vi "_check_error.vi"(8 "error in (no error)":errorcluster, 11 "VISA resource name":refnum<visa-resource-name>) -> (0 "error out":errorcluster, 3 "VISA resource name out":refnum<visa-resource-name>)   [LabVIEW 2015, in "Rohde&Schwarz CMXP Base.lvlib"]
doc: "This VI checks for an error by sending *STB? query to the instrument. If the bit 2 (0x04) is set, it sends multiple SYST:ERR? queries to the instrument until the error query is empty."
uses:
  <instrlib>/Rohde&Schwarz CMXP Base/Rohde&Schwarz CMXP Base.lvlib
  <instrlib>/Rohde&Schwarz CMXP Base/Private/rsidr_core.llb/type_Attribute.ctl
  <instrlib>/Rohde&Schwarz CMXP Base/Private/rsidr_core.llb/type_Attribute_Data_Type.ctl
  <instrlib>/Rohde&Schwarz CMXP Base/Private/rsidr_core.llb/type_ReadWriteAccess.ctl
  <instrlib>/Rohde&Schwarz CMXP Base/Private/rsidr_core.llb/rsidr_core.lvlib
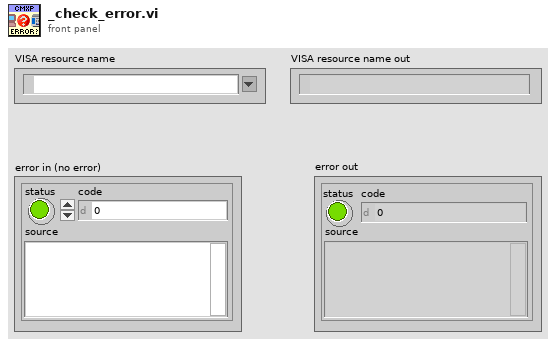
[diagram p1: front panel]
types:
  T1 = typedef "Rohde&Schwarz CMXP Base.lvlib/rsidr_core.lvlib/type_Attribute.ctl" = cluster{"Identifier":string, "Descriptive Name":string, "Data Type":T2, "Command":string, "Access":T3, "Range Table":string, "Read Callback":string, "Write Callback":string, "Supported Models":string, "Instrument Options":string, "Index":i32, "OPC Wait":bool, "No Status Check":bool, "Cache Only":bool}
  T2 = typedef "Rohde&Schwarz CMXP Base.lvlib/rsidr_core.lvlib/type_Attribute_Data_Type.ctl" = enum16{"Integer 32", "Double", "String", "Boolean", "None", "Integer 64", "RawString"}
  T3 = typedef "Rohde&Schwarz CMXP Base.lvlib/rsidr_core.lvlib/type_ReadWriteAccess.ctl" = enum16{"Read Only", "Write Only", "Read/Write"}
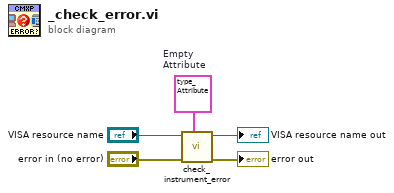
[diagram p0: block diagram]
diagram:
  w1 = T1 {"Identifier"="", "Descriptive Name"="", "Data Type"=enum."Integer 32", "Command"="", "Access"=enum."Read/Write", "Range Table"="", "Read Callback"="", "Write Callback"="", "Supported Models"="", "Instrument Options"="", "Index"=0, "OPC Wait"=FALSE, "No Status Check"=FALSE, "Cache Only"=FALSE}  # Empty Attribute
  n1 = call <instrlib>:"check_instrument_error.vi"("Attribute"=w1, "error in"="error in (no error)", "VISA resource name"="VISA resource name") -> ("error out"=→"error out":errorcluster, "VISA resource name out"=→"VISA resource name out":refnum<visa-resource-name>)  [unwired: 7 in]
